vi "GenerateAISharedVariables.vi"(8 "error in (no error)":errorcluster, 10 "ChannelNames":string[](array[string]), 11 "DeviceName":string) -> (0 "error out":errorcluster, 3 "Shared Library Path":path)   [LabVIEW 2013]
uses:
  SetListPrefs/SetListPrefs.lvclass/SetListPrefs.ctl
  Globals/PrefsGlobal.vi
  SetListPrefs/SetListPrefs.lvclass
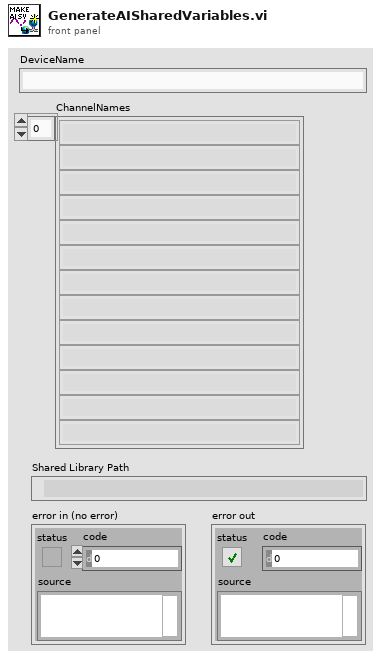
[diagram p1: front panel]
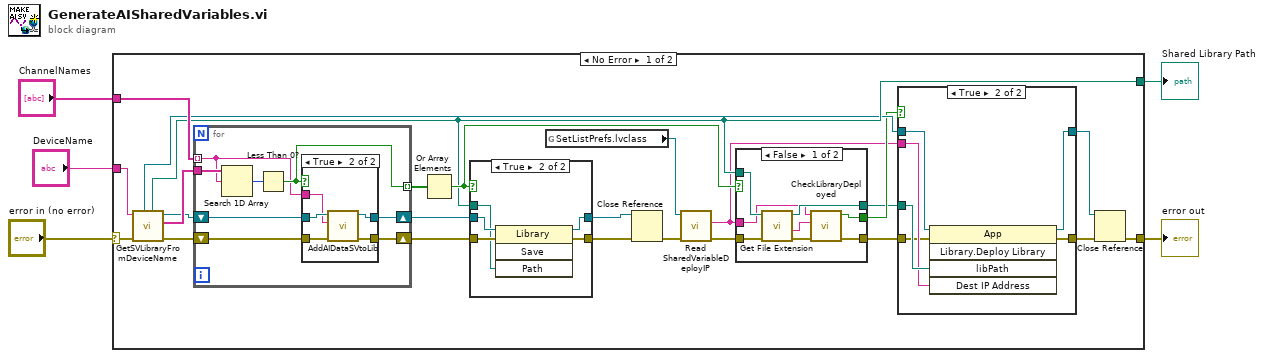
[diagram p0: block diagram]
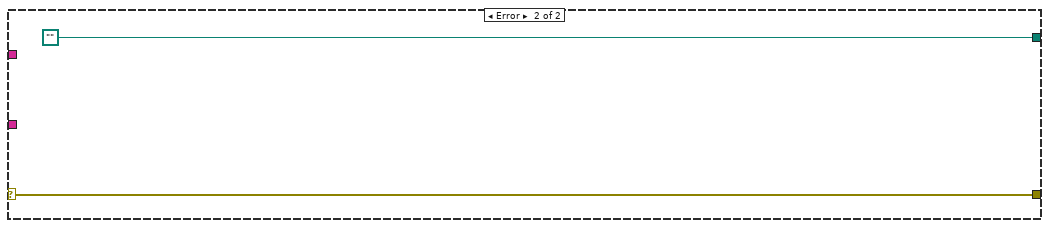
[diagram p6: hidden frame]
diagram:
  n1 = case shown="No Error" "error in (no error)" {
    selector: "error in (no error)" -> [w10 w71]
    tunnel: "ChannelNames" -> [w29 _]
    tunnel: "DeviceName" -> [w21 _]
    tunnel: [w18 path ""] -> w3
    tunnel: [w11 w71] -> w2
    frame No Error {
      n2 = call "GetSVLibraryFromDeviceName.vi"("error in (no error)"=w10, "DeviceName"=w21) -> ("error out"=w23:errorcluster, "Current Variables"=w20:string[], "Open Library Reference"=w19:refnum<vi>, "Library Path"=w18:path, "Application Reference"=w17:refnum<vi>)  [unwired: 5 in]
      n3 = for {
        tunnel: w29 -> [w56] mode=indexing
        tunnel: w20 -> [w63]
        shift-right: [w60] -> w28
        shift-left: w19 -> [w61]
        tunnel: [w59] -> w26 mode=indexing
        shift-right: [w58] -> w27
        shift-left: w23 -> [w57]
        n4 = Search 1D Array(1D array=w63, element=w56) -> (index of element=w62:i32)  [unwired: 1 in]
        n5 = Less Than 0?(x=w62) -> (x < 0?=w59:bool)
        n6 = case shown="True" w59 {
          tunnel: w61 -> [w65 w70]
          tunnel: [w65 w69] -> w60
          tunnel: [w64 w68] -> w58
          tunnel: w57 -> [w64 w67]
          tunnel: w56 -> [_ w66]
          frame False {
          }
          frame True {
            n7 = call "AddAIDataSVtoLib.vi"("error in (no error)"=w67, "Name"=w66, "Library in"=w70) -> ("error out"=w68:errorcluster, "Library out"=w69:refnum<vi>)  [unwired: 7 in]
          }
        }
      }
      n8 = Or Array Elements(Boolean array=w26) -> (logical OR=w22:bool)
      n9 = case shown="True" w22 {
        tunnel: w28 -> [w49 w55]
        tunnel: w27 -> [w50 w54]
        tunnel: [w50 w52] -> w24
        tunnel: [w49 w53] -> w25
        tunnel: w18 -> [_ w51]
        frame False {
        }
        frame True {
          n10 = invoke class="Library" method="Save"(reference=w55, error in=w54, "Path"=w51) -> (reference out=w53:refnum<vi>, error out=w52:errorcluster)  [unwired: 1 in, 2 out]
        }
      }
      n11 = global read "PrefsGlobal.vi" "SetListPrefs.lvclass"() -> (w9:refnum<class "SetListPrefs.lvclass">)
      n12 = Close Reference(reference=w25, error in (no error)=w24) -> (error out=w7:errorcluster)
      n13 = call "Read SharedVariableDeployIP.vi"("error in (no error)"=w7, "SetListPrefs in"=w9) -> ("error out"=w6:errorcluster, "SharedVariableDeployIP"=w8:string)  [unwired: 7 in, 1 out]
      n14 = case shown="False" w22 {
        selector: w22 -> [_ w48]
        tunnel: [w45 w48] -> w16
        tunnel: w6 -> [w43 w47]
        tunnel: [w44 w47] -> w15
        tunnel: w18 -> [w41 w46]
        tunnel: [w39 w46] -> w14
        tunnel: w8 -> [w38 _]
        frame False {
          n15 = call <vilib>:"Get File Extension.vi"("error in (no error)"=w43, "file"=w41) -> ("error out"=w42:errorcluster, "filename without extension"=w40:string, "dup file"=w39:path)  [unwired: 6 in, 1 out]
          n16 = call "CheckLibraryDeployed.vi"("error in (no error)"=w42, "Container Name"=w40, "Target IP"=w38) -> ("error out"=w44:errorcluster, "needsDeploy"=w45:bool)  [unwired: 7 in]
        }
        frame True {
        }
      }
      n17 = case shown="True" w16 {
        tunnel: w17 -> [w31 w37]
        tunnel: w15 -> [w30 w32]
        tunnel: w14 -> [_ w36]
        tunnel: [w31 w35] -> w13
        tunnel: [w30 w34] -> w12
        tunnel: w8 -> [_ w33]
        frame False {
        }
        frame True {
          n18 = invoke class="App" method="Library.Deploy Library"(reference=w37, error in=w32, "libPath"=w36, "Dest IP Address"=w33) -> (reference out=w35:refnum<vi>, error out=w34:errorcluster)  [unwired: 1 in, 3 out]
        }
      }
      n19 = Close Reference(reference=w13, error in (no error)=w12) -> (error out=w11:errorcluster)
    }
    frame Error {
    }
  }
  "Shared Library Path" <- w3
  "error out" <- w2
